vi "CamIndex.vi"(6 "index":i32, 8 "error in (no error)":errorcluster, 11 "MagAnalysis_Online in":refnum<class "MagAnalysis_Online.lvclass">) -> (0 "error out":errorcluster, 1 "Cam Cluster out 2":T2={"incident ANGLE COMPENSATION"=[], "dp/B [MeV/C/B]"=[], "charge compensation"=[], "Momentum [MeV/C]"=[], "energyDependence Input"=[], "pixel angle (y)"=[], "dp [MeV/C/] "=[], "angle 2Dfor spectrumj"=[], "dp [MeV/C] 2D"=[], "charge compensation 2D"=[], "Screen&Camera 2"={"Screen Orientation"="Regular", "Screen angle"="Flat", "Lens"=enum."FL1-f8x08", "Calibration (mm/pix)"=1.0}, "ROI info"={"npix-X"=0, "npix-Y"=0, "Left [pix]"=0.0, "Top [pix]"=0.0}, "Y 2D full angle"=[], "calib pixel"={"y1(pixel)"=[], "y2(pixel)"=[], "dp/B [MeV/C/B] (pixel)"=[], "energyDependence Input(pixel)"=[], "bending angle [deg](pixel)"=[], "total path(pixel)"=[], "pixel angle (y)(pixel)"=[], "energy dependence (pixel)"=[], "charge compensation (pixel)"=[], "Momentum [MeV/C](pixel)"=[], "angular compensation(pixel)"=[]}, "2D"={"dp"=[], "chargeCompensation"=[], "angle"=[], "Momentum"=[]}, "UserROI"={"Width"=0.0, "Hight"=0.0, "OffsetX"=0.0, "OffsetY"=0.0}, "final"={"X"=[], "xi"=[], "delta momentum"=0.0, "Y"=[], "yi"=[], "angle (Y)"=[], "delta angle"=0.0, "scale delta angle"=0.0, "intraX"=0.0, "intraY"=0.0, "mask"=[]}, "B[T]"=0.0, "index"=0.0}, 2 "spec cluster":T1, 3 "z":dbl[][](array[numeric]), 7 "time":u32)   [LabVIEW 2020, in "MagAnalysis_Online.lvclass"]
uses:
  MagAnalysis_Online.lvclass
  calib_Sub_Typdef.ctl
  ScreenCam2_TypDEf.ctl
  CamAndObj_TypDEf.ctl
  ROIInfo_TypDef.ctl
  calibPixel.ctl
  2DTypDef.ctl
  CamRoiTypDef.ctl
  finalCalibTypdef.ctl
  specCluster_Typdef.ctl
  specClustercommandTypdef.ctl
  MagAnalysis_Online.lvclass/MagAnalysis_Online.ctl
  reshapeArrayCommand_TypDEf.ctl
panel:
  out "time:spec":u32
  out "time:cliab":u32
  out "FGV":u32
  out "time: AllProc":u32
  out "time":u32
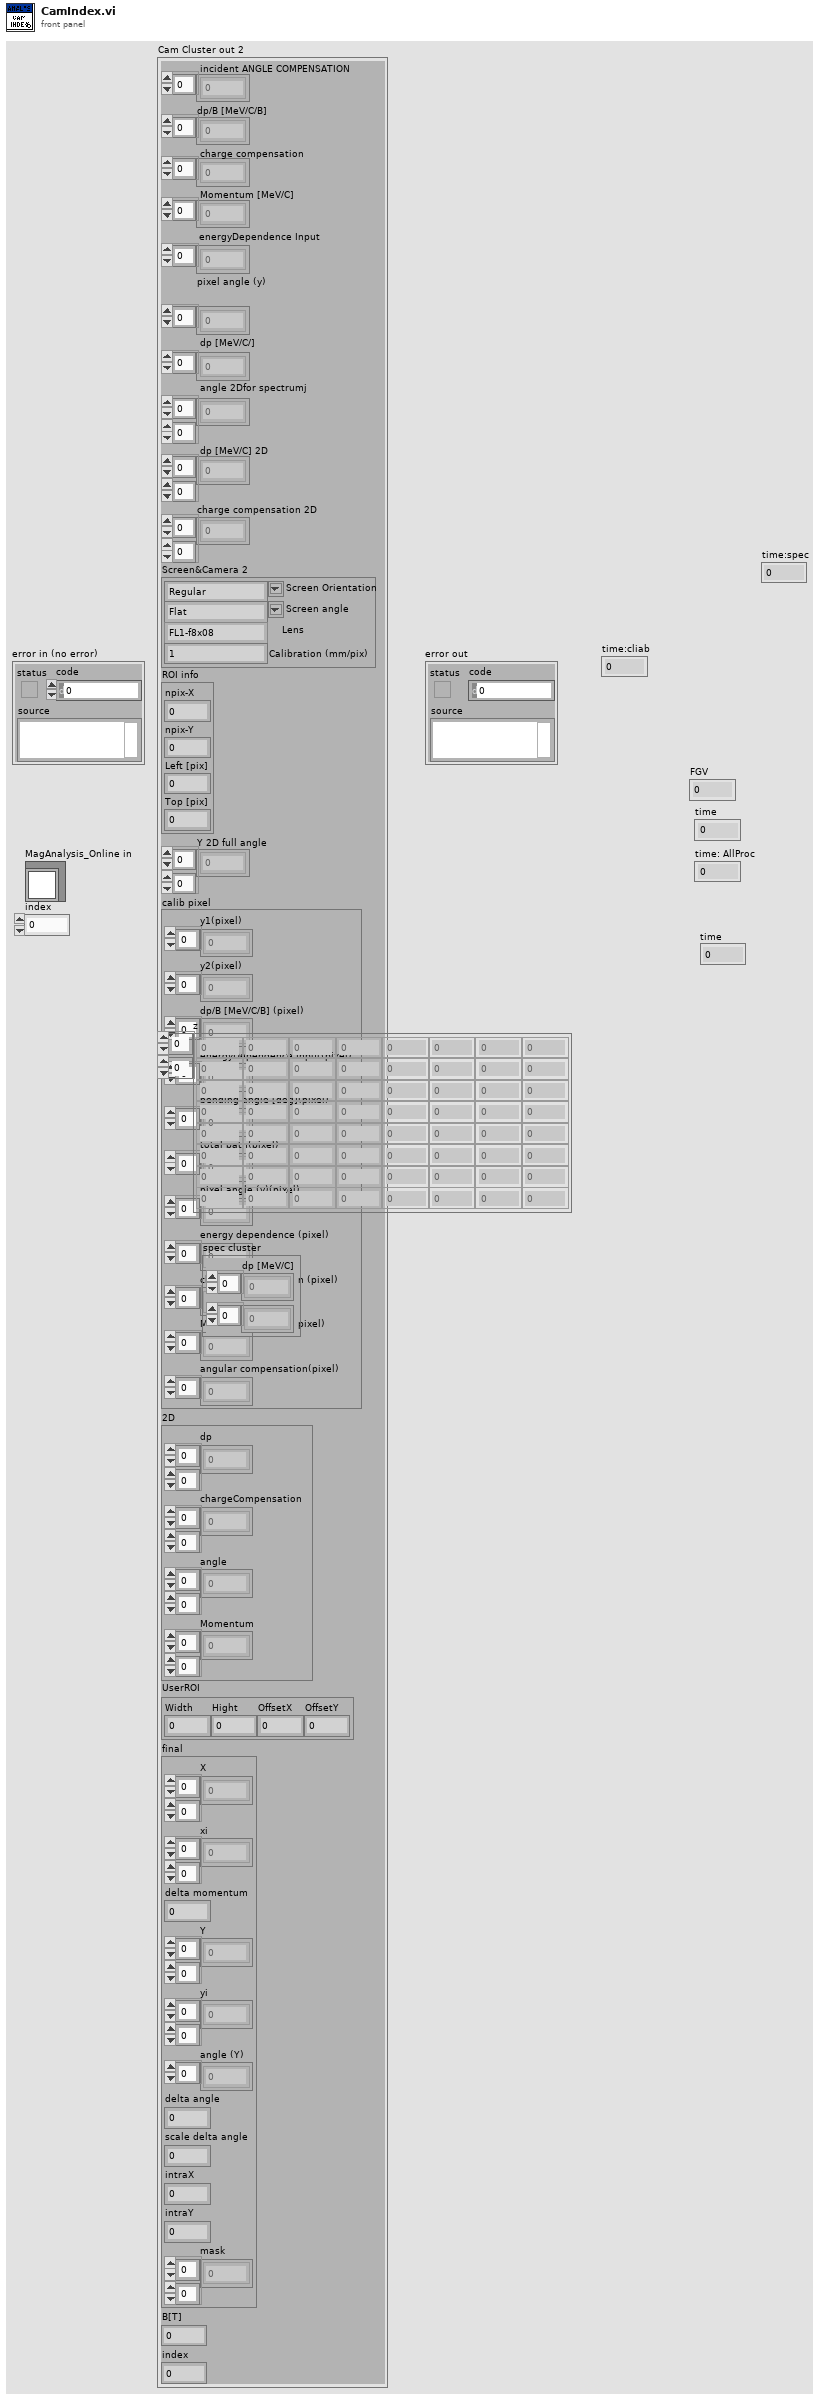
[diagram p1: front panel]
types:
  T1 = typedef "specCluster_Typdef.ctl" = cluster{"dp [MeV/C]":dbl[], dbl[]}
  T2 = typedef "calib_Sub_Typdef.ctl" = cluster{"incident ANGLE COMPENSATION":dbl[], "dp/B [MeV/C/B]":dbl[], "charge compensation":dbl[], "Momentum [MeV/C]":dbl[], "energyDependence Input":dbl[], "pixel angle (y)":dbl[], "dp [MeV/C/] ":dbl[], "angle 2Dfor spectrumj":dbl[][], "dp [MeV/C] 2D":dbl[][], "charge compensation 2D":dbl[][], "Screen&Camera 2":T3, "ROI info":T5, "Y 2D full angle":dbl[][], "calib pixel":T6, "2D":T7, "UserROI":T8, "final":T9, "B[T]":dbl, "index":dbl}
  T3 = typedef "ScreenCam2_TypDEf.ctl" = cluster{"Screen Orientation":string, "Screen angle":string, "Lens":T4, "Calibration (mm/pix)":dbl}
  T4 = typedef "CamAndObj_TypDEf.ctl" = enum16{"FL1-f8x08", "FL1-f8x06", "FL1-f8", "ch300-f50", "FL2G-f8", "FL3M14-f8", "FL3M14-f8x08", "FL3M14-f8x08(2x2)"}
  T5 = typedef "ROIInfo_TypDef.ctl" = cluster{"npix-X":i32, "npix-Y":i32, "Left [pix]":dbl, "Top [pix]":dbl}
  T6 = typedef "calibPixel.ctl" = cluster{"y1(pixel)":dbl[], "y2(pixel)":dbl[], "dp/B [MeV/C/B] (pixel)":dbl[], "energyDependence Input(pixel)":dbl[], "bending angle [deg](pixel)":dbl[], "total path(pixel)":dbl[], "pixel angle (y)(pixel)":dbl[], "energy dependence (pixel)":dbl[], "charge compensation (pixel)":dbl[], "Momentum [MeV/C](pixel)":dbl[], "angular compensation(pixel)":dbl[]}
  T7 = typedef "2DTypDef.ctl" = cluster{"dp":dbl[][], "chargeCompensation":dbl[][], "angle":dbl[][], "Momentum":dbl[][]}
  T8 = typedef "CamRoiTypDef.ctl" = cluster{"Width":dbl, "Hight":dbl, "OffsetX":dbl, "OffsetY":dbl}
  T9 = typedef "finalCalibTypdef.ctl" = cluster{"X":dbl[][], "xi":dbl[][], "delta momentum":dbl, "Y":dbl[][], "yi":dbl[][], "angle (Y)":dbl[], "delta angle":dbl, "scale delta angle":dbl, "intraX":dbl, "intraY":dbl, "mask":dbl[][]}
  T10 = typedef "specClustercommandTypdef.ctl" = enum16{"init", "addCluster", "read", "clear"}
  T11 = typedef "reshapeArrayCommand_TypDEf.ctl" = enum16{"init array", "addImage", "read", "init resolution"}
  T12 = typedef "MagAnalysis_Online.lvclass/analysis_data_typdef.ctl" = cluster{"cam0":T13, "cam1":T13, "cam2":T13, "cam3":T13}
  T13 = typedef "IMAQ Image.ctl" = refnum<image>
  T14 = typedef "bgImages_tyudef.ctl" = cluster{"cam 0":T13, "cam 1":T13, "cam 2":T13, "cam 3":T13}
  T15 = typedef "reshapeINfo_TypDef.ctl" = cluster{"emptyImageArray":dbl[], "max Y size":i32, "X size":i32, "number of cam":i32, "emptyZArrayforreshape":T16}
  T16 = typedef "emptyArray_TYpDEf.ctl" = cluster{"Cam 0":T17, "Cam 1":T17, "Cam 2":T17, "Cam 3":T17}
  T17 = typedef "emptyArrayCamX_TypDef.ctl" = cluster{"1":dbl[][], "2":dbl[][]}
  T18 = cluster{"S 0":i32[][], "S 1":i32[][], "S 2":i32[][], "S 3":i32[][]}
  T19 = typedef "Calib_Typdef.ctl" = cluster{"cam 0":T2, "cam 1":T2, "cam 2":T2, "cam 3":T2}
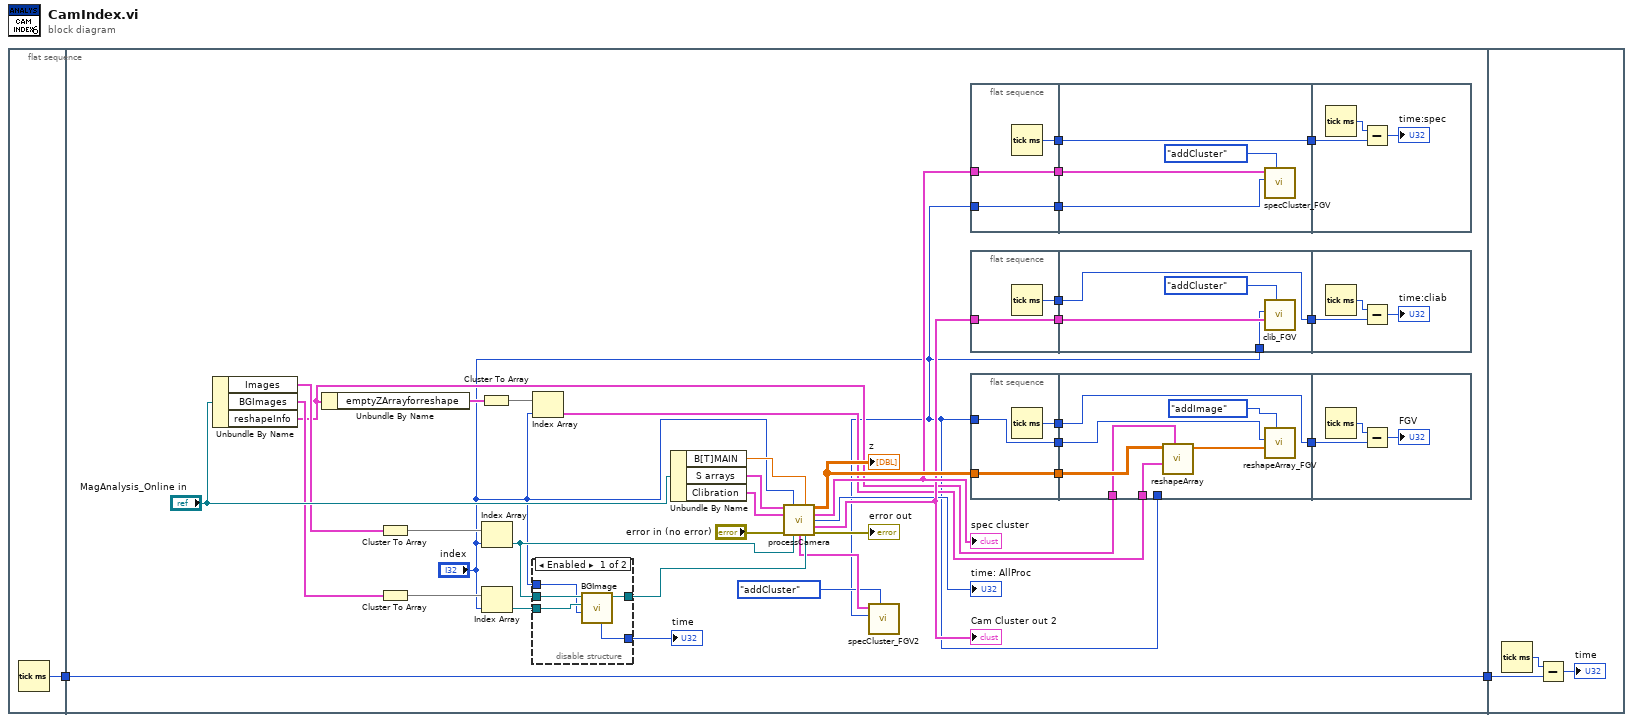
[diagram p0: block diagram]
diagram:
  n1 = flat-sequence {
    tunnel: [w3] -> w2
    tunnel: w2 -> [w25]
    tunnel: [w25] -> w1
    tunnel: w1 -> [w79]
    frame #0 {
      n2 = Tick Count (ms)() -> (millisecond timer value=w3:u32)
    }
    frame #1 {
      n3 = Unbundle By Name("MagAnalysis_Online in") -> ("Images"=w31:T12, "BGImages"=w30:T14, "reshapeInfo"=w12:T15)
      n4 = Unbundle By Name(w12) -> ("emptyZArrayforreshape"=w11:T16)
      n5 = Cluster To Array(cluster=w31) -> (array=w38:T13[])
      n6 = Cluster To Array(cluster=w30) -> (array=w39:T13[])
      n7 = Cluster To Array(cluster=w11) -> (array=w10:T17[])
      n8 = Index Array(array=w38, index="index") -> (element=w34:T13)
      n9 = Index Array(array=w39, index="index") -> (element=w40:T13)
      n10 = Index Array(array=w10, index="index") -> (element=w9:T17)
      n11 = disable-structure shown="Enabled" {
        disable-tunnel: w40 -> [w45 w46]
        disable-tunnel: [w44 w46] -> w35
        disable-tunnel: w34 -> [w43 _]
        disable-tunnel: "index" -> [w42 _]
        disable-tunnel: [w41 _] -> w26
        frame Enabled {
          n12 = call "BGImage.vi"("index"=w42, "BG"=w45, "Image"=w43) -> ("Refnum out"=w44:T13, "time"=w41:u32)  [unwired: 7 in]
        }
        frame Disabled {
        }
      }
      "time" <- w26
      n13 = Unbundle By Name("MagAnalysis_Online in") -> ("B[T]MAIN"=w33:dbl, "S arrays"=w36:T18, "Clibration"=w37:T19)
      n14 = call "processCamera.vi"("S arrays"=w36, "index"="index", "B [T]"=w33, "Clibration"=w37, "error in (no error)"="error in (no error)", "image in"=w34, "bg in"=w35) -> ("z"=w29:dbl[][], "spec cluster"=w28:cluster{"dp [MeV/C]":dbl[], dbl[]}, "time: AllProc"=→"time: AllProc":u32, "Cam Cluster out 2"=w27:T2, "Sum Y"=w6:cluster{"Ramp Pattern":dbl[], dbl[]}, "error out"=→"error out":errorcluster)  [unwired: 3 in]
      "Cam Cluster out 2" <- w27
      "spec cluster" <- w28
      "z" <- w29
      n15 = call "specCluster_FGV2.vi"("command"=specClustercommandTypdef."addCluster", "index"="index", "spec cluster"=w6) -> ()  [unwired: 7 in, 2 out]
      n16 = flat-sequence {
        tunnel: "index" -> [w48]
        tunnel: w28 -> [w49]
        tunnel: [w49] -> w16
        tunnel: [w48] -> w15
        tunnel: [w47] -> w13
        tunnel: w16 -> [w53]
        tunnel: w15 -> [w52]
        tunnel: [w50] -> w14
        tunnel: w13 -> [w50]
        tunnel: w14 -> [w54]
        frame #0 {
          n17 = Tick Count (ms)() -> (millisecond timer value=w47:u32)
        }
        frame #1 {
          n18 = call "specCluster_FGV.vi"("command"=specClustercommandTypdef."addCluster", "index"=w52, "spec cluster"=w53) -> ()  [unwired: 7 in, 2 out]
        }
        frame #2 {
          n19 = Tick Count (ms)() -> (millisecond timer value=w56:u32)
          n20 = Subtract(x=w56, y=w54) -> (x-y=→"time:spec":u32)
        }
      }
      n21 = flat-sequence {
        tunnel: w27 -> [w58]
        tunnel: [w58] -> w19
        tunnel: [w57] -> w18
        tunnel: "index" -> [w61]
        tunnel: w19 -> [w62]
        tunnel: w18 -> [w59]
        tunnel: [w59] -> w17
        tunnel: w17 -> [w63]
        frame #0 {
          n22 = Tick Count (ms)() -> (millisecond timer value=w57:u32)
        }
        frame #1 {
          n23 = call "clib_FGV.vi"("command"=specClustercommandTypdef."addCluster", "Cam Cluster out 2"=w62, "index"=w61) -> ()  [unwired: 7 in, 2 out]
        }
        frame #2 {
          n24 = Tick Count (ms)() -> (millisecond timer value=w64:u32)
          n25 = Subtract(x=w64, y=w63) -> (x-y=→"time:cliab":u32)
        }
      }
      n26 = flat-sequence {
        tunnel: "index" -> [w67]
        tunnel: w29 -> [w68]
        tunnel: [w68] -> w23
        tunnel: [w67] -> w22
        tunnel: [w66] -> w21
        tunnel: w23 -> [w75]
        tunnel: w22 -> [w74]
        tunnel: w21 -> [w72]
        tunnel: [w72] -> w20
        tunnel: w12 -> [w70]
        tunnel: w9 -> [w69]
        tunnel: "index" -> [_]
        tunnel: w20 -> [w76]
        frame #0 {
          n27 = Tick Count (ms)() -> (millisecond timer value=w66:u32)
        }
        frame #1 {
          n28 = call "reshapeArray.vi"("reshapeInfo"=w70, "element"=w69, "z"=w75) -> ("reshaped array"=w71:dbl[])  [unwired: 8 in]
          n29 = call "reshapeArray_FGV.vi"("command"=reshapeArrayCommand_TypDEf."addImage", "reshapedArray CamX"=w71, "index"=w74) -> ()  [unwired: 7 in, 2 out]
        }
        frame #2 {
          n30 = Tick Count (ms)() -> (millisecond timer value=w77:u32)
          n31 = Subtract(x=w77, y=w76) -> (x-y=→"FGV":u32)
        }
      }
    }
    frame #2 {
      n32 = Tick Count (ms)() -> (millisecond timer value=w81:u32)
      n33 = Subtract(x=w81, y=w79) -> (x-y=→"time":u32)
    }
  }
